vi "TDP.vi"(10 "Current Robot":T1, 11 "Al Input":T3) -> (3 "Output Robot":T1)   [LabVIEW 2016]
uses:
  Core/AI Input.ctl
  Core/AI Robot.ctl
  Functions Enum.ctl
  Core/AI Ball.ctl
  Core/Field Size.ctl
  Core/AI Judge.ctl
  Command Enum.ctl
  <vilib>/Analysis/_algsub.llb/Real Vector Norm.vi
  <vilib>/Analysis/NI_AALPro.lvlib
panel:
  out "Angulo":dbl
  in  "Closest Robot":T1
  in  "Closest Distance":dbl=999999999.0 format="%#_13g"
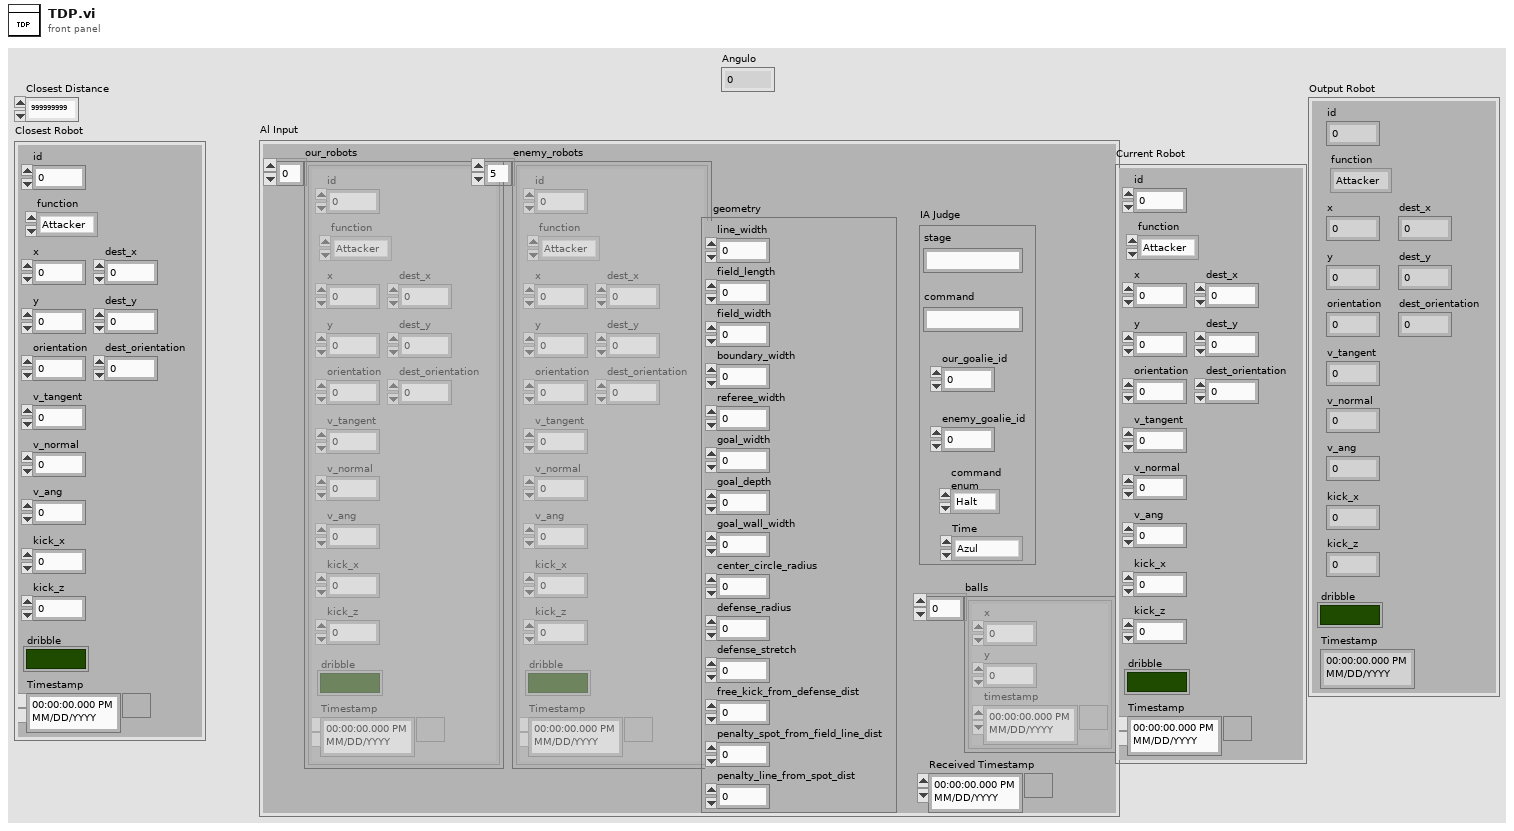
[diagram p1: front panel]
types:
  T1 = typedef "AI Robot.ctl" = cluster{"id":u32, "function":T2, "x":dbl, "y":dbl, "orientation":dbl, "v_tangent":dbl, "v_normal":dbl, "v_ang":dbl, "kick_x":dbl, "kick_z":dbl, "dribble":bool, "Timestamp":timestamp, "dest_x":dbl, "dest_y":dbl, "dest_orientation":dbl}
  T2 = typedef "Functions Enum.ctl" = enum16{"Attacker", "Goalie", "Defender", "Goto 0", "Dummy", "TDP"}
  T3 = typedef "AI Input.ctl" = cluster{"our_robots":T1[], "enemy_robots":T1[], "balls":T4[], "geometry":T5, "IA Judge":T6, "Received Timestamp":timestamp}
  T4 = typedef "AI Ball.ctl" = cluster{"x":dbl, "y":dbl, "timestamp":timestamp}
  T5 = typedef "Field Size.ctl" = cluster{"line_width":u32, "field_length":u32, "field_width":u32, "boundary_width":u32, "referee_width":u32, "goal_width":u32, "goal_depth":u32, "goal_wall_width":u32, "center_circle_radius":u32, "defense_radius":u32, "defense_stretch":u32, "free_kick_from_defense_dist":u32, "penalty_spot_from_field_line_dist":u32, "penalty_line_from_spot_dist":u32}
  T6 = typedef "AI Judge.ctl" = cluster{"stage":string, "command":string, "our_goalie_id":dbl, "enemy_goalie_id":dbl, "command\nenum":T7, "Time":enum16{"Azul", "Amarelo"}}
  T7 = typedef "Command Enum.ctl" = enum16{"Halt", "Stop", "Force Start", "PKA Normal Start", "Prepare Kickoff Ally", "PKE Normal Start", "Prepare Kickoff Enemy", "Prepare Penalty Ally", "PPA Normal Start", "Prepare Penalty Enemy", "PPE Normal Start", "Direct Free Enemy", "Direct Free Ally", "Indirect Free Enemy", "Indirect Free Ally", "Timeout Enemy", "Timeout Ally", "Goal Enemy", "Goal Ally", "Ball Placement Enemy", "Ball Placement Ally", "None"}
  T8 = cluster{"id":bool, "function":bool, "x":bool, "y":bool, "orientation":bool, "v_tangent":bool, "v_normal":bool, "v_ang":bool, "kick_x":bool, "kick_z":bool, "dribble":bool, "Timestamp":bool, "dest_x":bool, "dest_y":bool, "dest_orientation":bool}
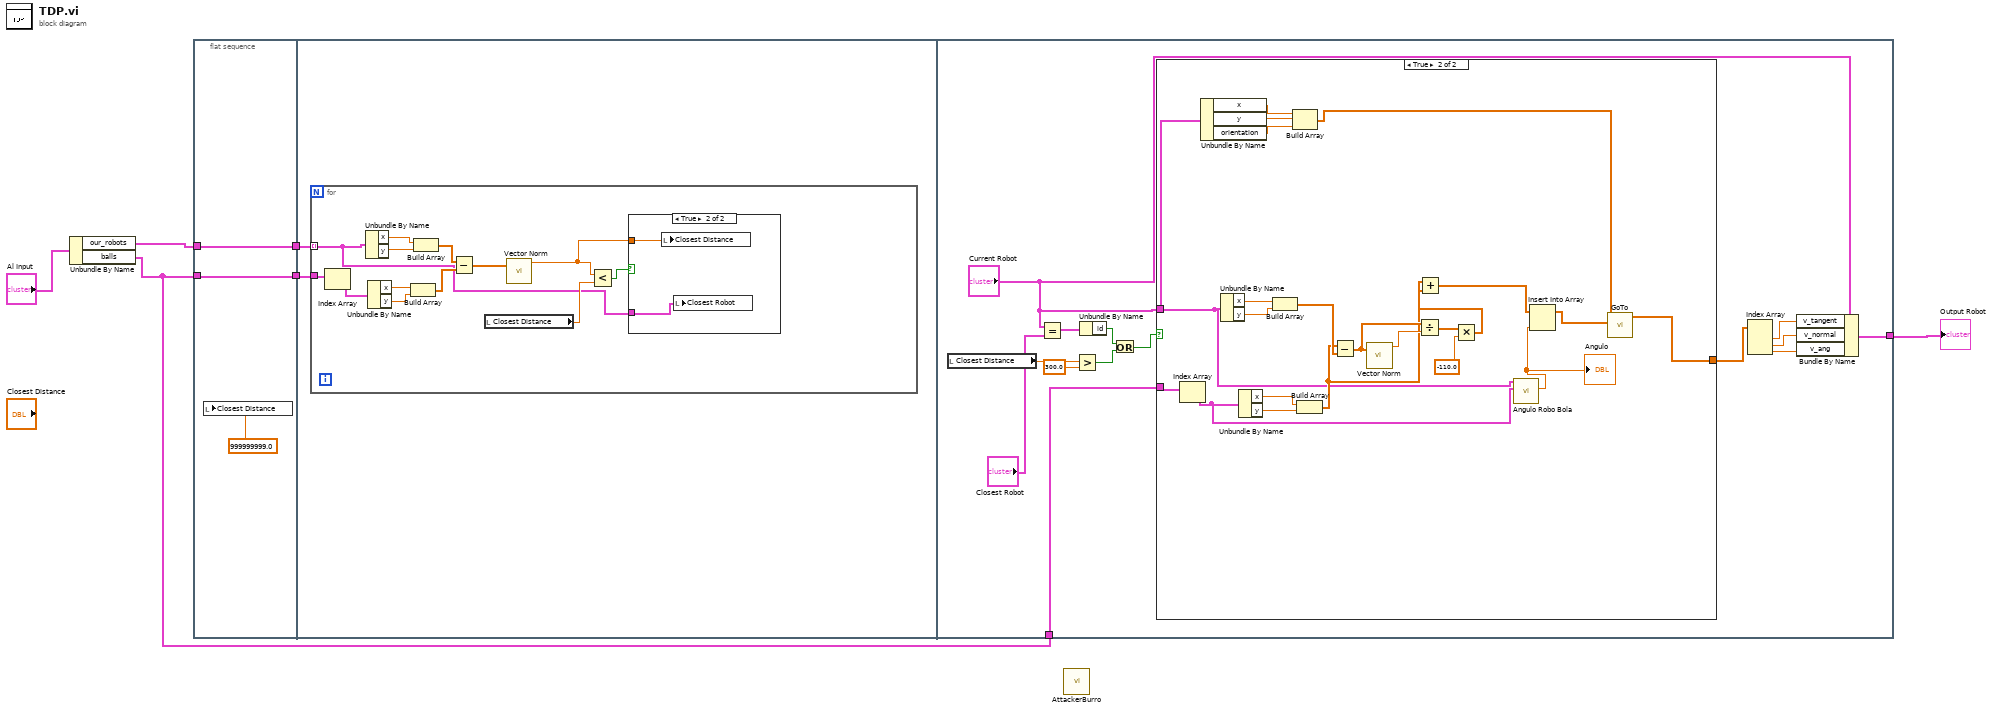
[diagram p0: block diagram]
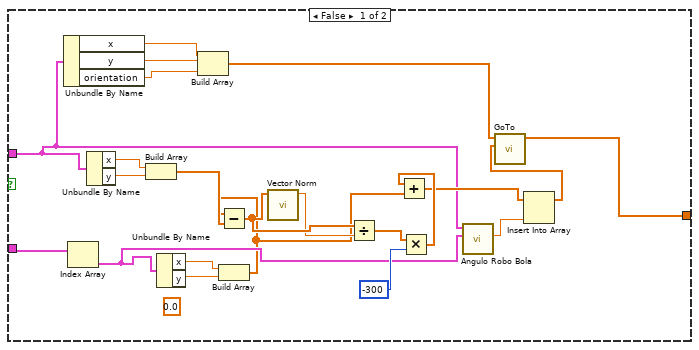
[diagram p3: hidden frame]
diagram:
  n1 = Unbundle By Name("Al Input") -> ("our_robots"=w6:T1[], "balls"=w4:T4[])
  n2 = flat-sequence {
    tunnel: w4 -> [w8]
    tunnel: w6 -> [w9]
    tunnel: [w9] -> w2
    tunnel: [w8] -> w1
    tunnel: w2 -> [w11]
    tunnel: w1 -> [w10]
    tunnel: w4 -> [w38]
    tunnel: [w32] -> w3
    frame #0 {
      n3 = local write "Closest Distance"(999999999.0 ("Closest Distance")) -> ()
    }
    frame #1 {
      n4 = for {
        tunnel: w11 -> [w12] mode=indexing
        tunnel: w10 -> [w24]
        n5 = Index Array(array=w24) -> (element=w23:T4)  [unwired: 1 in]
        n6 = Unbundle By Name(w12) -> ("x"=w22:dbl, "y"=w21:dbl)
        n7 = Unbundle By Name(w23) -> ("x"=w20:dbl, "y"=w19:dbl)
        n8 = Build Array(w20, w19) -> (w17:dbl[])
        n9 = Build Array(w22, w21) -> (w18:dbl[])
        n10 = Subtract(x=w18, y=w17) -> (x-y=w16:dbl[])
        n11 = local read "Closest Distance"() -> (w15:dbl)
        n12 = call-poly <vilib>:"Vector Norm.vi"("Input Vector"=w16) -> ("norm"=w13:dbl)  [unwired: 9 in, 1 out]
        n13 = Less?(x=w13, y=w15) -> (x < y?=w14:bool)
        n14 = case shown="True" w14 {
          tunnel: w13 -> [_ w26]
          tunnel: w12 -> [_ w25]
          frame False {
          }
          frame True {
            n15 = local write "Closest Distance"(w26) -> ()
            n16 = local write "Closest Robot"(w25) -> ()
          }
        }
      }
    }
    frame #2 {
      n17 = local read "Closest Distance"() -> (w31:dbl)
      n18 = Equal?(x="Current Robot", y="Closest Robot") -> (x = y?=w39:T8)
      n19 = Greater?(x=w31, y=300.0) -> (0:w28:bool)
      n20 = Unbundle By Name(w39) -> ("id"=w29:bool)
      n21 = Or(x=w29, y=w28) -> (x .or. y?=w27:bool)
      n22 = case shown="True" w27 {
        tunnel: w38 -> [w62 w84]
        tunnel: "Current Robot" -> [w48 w67]
        tunnel: [w43 w77] -> w36
        frame False {
          (unwired) 0.0 ("element")
          n23 = Unbundle By Name(w48) -> ("x"=w47:dbl, "y"=w46:dbl, "orientation"=w45:dbl)
          n24 = Index Array(array=w62) -> (element=w50:T4)  [unwired: 1 in]
          n25 = Unbundle By Name(w48) -> ("x"=w61:dbl, "y"=w60:dbl)
          n26 = Build Array(w61, w60) -> (w56:dbl[])
          n27 = Unbundle By Name(w50) -> ("x"=w59:dbl, "y"=w58:dbl)
          n28 = Build Array(w47, w46, w45) -> (w44:dbl[])
          n29 = Build Array(w59, w58) -> (w41:dbl[])
          n30 = Subtract(x=w41, y=w56) -> (x-y=w57:dbl[])
          n31 = call-poly <vilib>:"Vector Norm.vi"("Input Vector"=w57) -> ("norm"=w42:dbl)  [unwired: 9 in, 1 out]
          n32 = Divide(x=w57, y=w42) -> (x/y=w55:dbl[])
          n33 = Multiply(x=w55, y=-300) -> (x*y=w53:dbl[])
          n34 = Add(x=w53, y=w41) -> (x+y=w52:dbl[])
          n35 = call "Angulo Robo Bola.vi"("Ball"=w50, "Robot"=w48) -> ("Angulo"=w51:dbl)  [unwired: 9 in]
          n36 = Insert Into Array(array=w52, new element=w51) -> (w49:dbl[])  [unwired: 1 in]
          n37 = call "GoTo.vi"("Target"=w49, "Position"=w44) -> ("Output\nVelocity"=w43:dbl[])  [unwired: 9 in]
        }
        frame True {
          n38 = Index Array(array=w84) -> (element=w66:T4)  [unwired: 1 in]
          n39 = Unbundle By Name(w67) -> ("x"=w81:dbl, "y"=w80:dbl, "orientation"=w79:dbl)
          n40 = Unbundle By Name(w67) -> ("x"=w76:dbl, "y"=w75:dbl)
          n41 = Unbundle By Name(w66) -> ("x"=w83:dbl, "y"=w82:dbl)
          n42 = Build Array(w76, w75) -> (w74:dbl[])
          n43 = Build Array(w81, w80, w79) -> (w78:dbl[])
          n44 = Build Array(w83, w82) -> (w71:dbl[])
          n45 = Subtract(x=w71, y=w74) -> (x-y=w73:dbl[])
          n46 = call-poly <vilib>:"Vector Norm.vi"("Input Vector"=w73) -> ("norm"=w72:dbl)  [unwired: 9 in, 1 out]
          n47 = Divide(x=w73, y=w72) -> (x/y=w70:dbl[])
          n48 = Multiply(x=w70, y=-110.0) -> (x*y=w68:dbl[])
          n49 = Add(x=w71, y=w68) -> (x+y=w65:dbl[])
          n50 = call "Angulo Robo Bola.vi"("Ball"=w66, "Robot"=w67) -> ("Angulo"=w64:dbl)  [unwired: 9 in]
          "Angulo" <- w64
          n51 = Insert Into Array(array=w65, new element=w64) -> (w63:dbl[])  [unwired: 1 in]
          n52 = call "GoTo.vi"("Target"=w63, "Position"=w78) -> ("Output\nVelocity"=w77:dbl[])  [unwired: 9 in]
        }
      }
      n53 = Index Array(array=w36) -> (element #1=w35:dbl, element #2=w34:dbl, element #3=w33:dbl)  [unwired: 3 in]
      n54 = Bundle By Name(cluster="Current Robot", "v_tangent"=w35, "v_normal"=w34, "v_ang"=w33) -> (w32:T1)
    }
  }
  n55 = call "AttackerBurro.vi"() -> ()  [unwired: 11 in, 1 out]
  "Output Robot" <- w3
